vi "Set Measurement Mode.vi"(8 "error in (no error)":errorcluster, 10 "Measurement Mode":T1, 11 "2936r in":refnum<class "2936r.lvclass">) -> (0 "error out":errorcluster, 3 "2936r out":refnum<class "2936r.lvclass">)   [LabVIEW 2018, in "2936r.lvlib" / "2936r.lvclass"]
uses:
  2936r.lvclass
  PPLs/Optical Power Meter/Optical Power Meter.lvlibp/Custom Controls/Measurement Mode.ctl
  2936r.lvclass/2936r.ctl
  PPLs/Optical Power Meter/Optical Power Meter.lvlibp
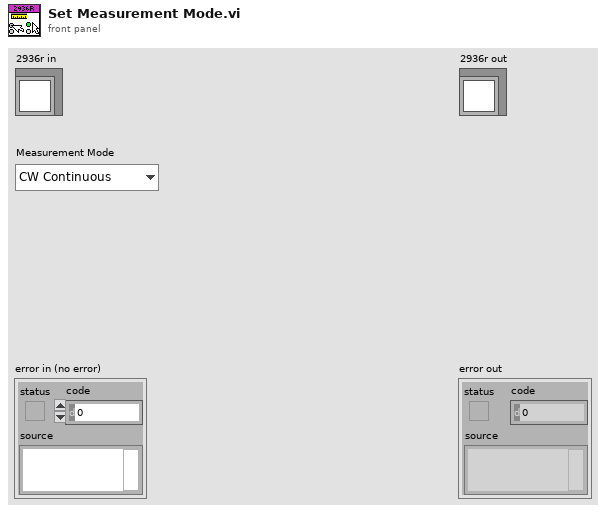
[diagram p1: front panel]
types:
  T1 = typedef "Optical Power Meter.lvlibp/Measurement Mode.ctl" = enum16{"CW Continuous", "CW Single", "CW Integrate", "PK-PK Continuous", "PK-PK Single", "RMS"}
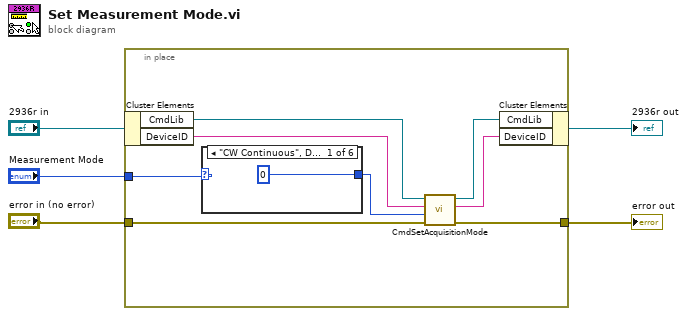
[diagram p0: block diagram]
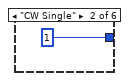
[diagram p2: hidden frame]
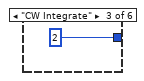
[diagram p3: hidden frame]
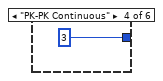
[diagram p4: hidden frame]
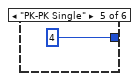
[diagram p5: hidden frame]
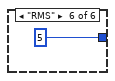
[diagram p6: hidden frame]
diagram:
  n1 = in-place {
    in-place-border: [w10] -> w3
    in-place-border: "error in (no error)" -> [w11]
    in-place-border: "Measurement Mode" -> [w9]
    n2 = in-place-cluster #1("2936r in") -> ("CmdLib"=w13:refnum<k24>, "DeviceID"=w12:string)
    n3 = case shown="\"CW Continuous\", Default" w9 {
      tunnel: [0 1 2 3 4 5] -> w8
      frame "CW Continuous", Default {
      }
      frame "CW Single" {
      }
      frame "CW Integrate" {
      }
      frame "PK-PK Continuous" {
      }
      frame "PK-PK Single" {
      }
      frame "RMS" {
      }
    }
    n4 = call <instrlib>:"CmdSetAcquisitionMode.vi"("error in (no error)"=w11, "Mode"=w8, "Device Key In"=w12, "CmdLib In"=w13) -> ("error out"=w10:errorcluster, "Device Key Out"=w6:string, "CmdLib Out"=w7:refnum<k24>)  [unwired: 4 in, 1 out]
    n5 = in-place-cluster #1("CmdLib"=w7, "DeviceID"=w6) -> (→"2936r out":refnum<class "2936r.lvclass">)
  }
  "error out" <- w3
